vi "ALTS-2015 OPC To URL.vi"(3 "Update rate (100 ms)":u32=100, 4 "Item Name":string, 5 "Server Name":string, 6 "Hostname (blank)":string) -> (0 "URL":string)   [LabVIEW 2013]
panel:
  # "Create an OPC URL from Several Inputs"
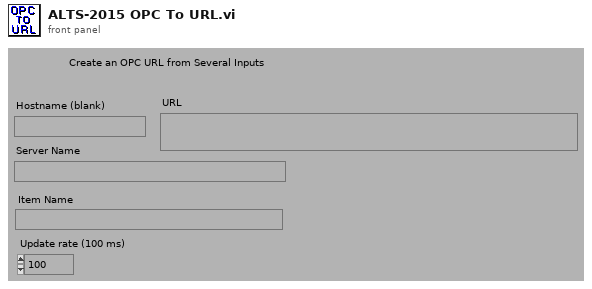
[diagram p1: front panel]
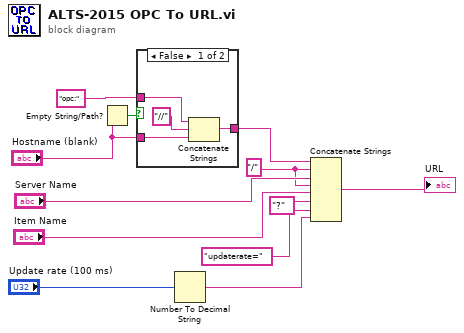
[diagram p0: block diagram]
diagram:
  w7 = "/"
  n1 = Empty String/Path?(string/path="Hostname (blank)") -> (empty?=w12:bool)
  n2 = case shown="False" w12 {
    tunnel: "opc:" -> [w16 w17]
    tunnel: [w15 w17] -> w9
    tunnel: "Hostname (blank)" -> [w14 _]
    frame False {
      n3 = Concatenate Strings(w16, "//" ("Hostname (blank)"), w14) -> (w15:string)
    }
    frame True {
    }
  }
  n4 = Number To Decimal String(number="Update rate (100 ms)") -> (decimal integer string=w4:string)  [unwired: 1 in]
  n5 = Concatenate Strings(w9, w7, "Server Name", w7, "Item Name", "?", "updaterate=", w4) -> (→"URL":string)
